vi "DHE_DRV_feedBuffers.vi"(10 "bufsize":u64) -> (0 "error out":errorcluster)   [LabVIEW 2016]
uses:
  c/lib/libarcDHE.so
panel:
  out "error out 2":errorcluster
  in  "stop":bool
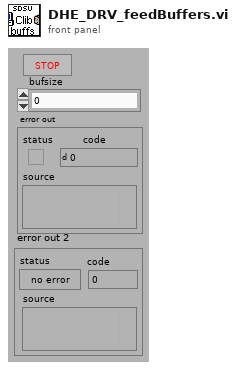
[diagram p1: front panel]
types:
  T1 = cluster{"Name":string, "size (bytes)":u32, "pointer":u32, "Lock":bool}
  T2 = cluster{"Name":string, "size (bytes)":u64, "pointer":u64, "Lock":bool}
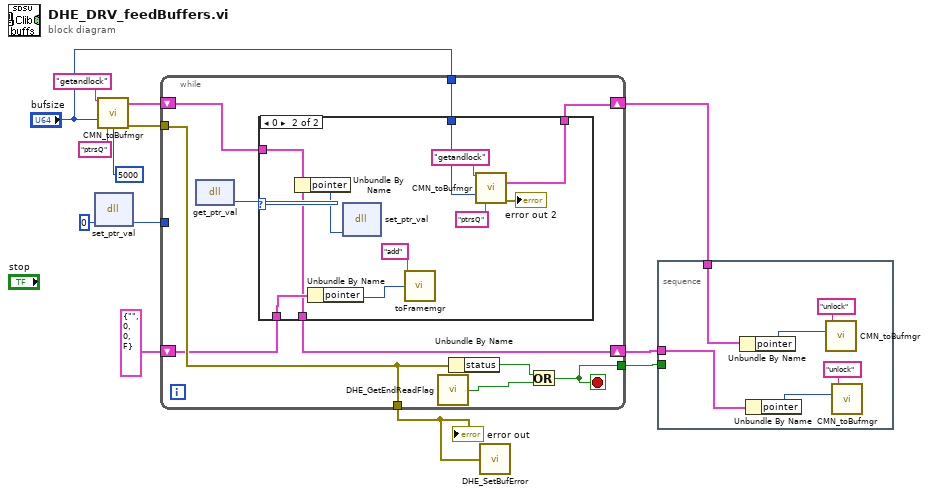
[diagram p0: block diagram]
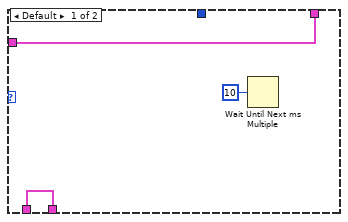
[diagram p2: hidden frame]
diagram:
  n1 = dll-call lib="home/simager/panview/PAN/Modules/SDSU/private/c/lib/libarcDHE.so" fn="set_ptr_val"("ptr"=u64 0) -> ("ptr"=w9:u64)  [unwired: 3 in, 3 out]
  n2 = call "CMN_toBufmgr.vi"("command"="getandlock", "bufsize"="bufsize", "responseQ"="ptrsQ", "ms timeout (-1)"=5000) -> ("buffer"=w11:T2, "error out"=w4:errorcluster)  [unwired: 4 in, 6 out]
  n3 = while {
    tunnel: [w17] -> w1
    tunnel: w4 -> [w17]
    tunnel: [w19] -> w7
    tunnel: "bufsize" -> [w20]
    tunnel: w9 -> [_]
    shift-left: T1 {"Name"="", "size (bytes)"=0, "pointer"=0, "Lock"=FALSE} ("buffer") -> [w16]
    shift-right: [w15] -> w6
    shift-left: w11 -> [w22]
    shift-right: [w21] -> w3
    stop <- w19 stop-if-true
    n4 = dll-call lib="home/simager/panview/PAN/Modules/SDSU/private/c/lib/libarcDHE.so" fn="get_ptr_val"() -> ("return type"=w23:u64)  [unwired: 3 in, 2 out]
    n5 = case shown="0" w23 {
      tunnel: w22 -> [w25 w28]
      tunnel: [w25 w33] -> w21
      tunnel: w20 -> [_ w30]
      tunnel: w16 -> [w24 w29]
      tunnel: [w24 w28] -> w15
      frame Default {
        n6 = Wait Until Next ms Multiple(millisecond multiple=u32 10) -> ()  [unwired: 1 out]
      }
      frame 0 {
        n7 = Unbundle By Name(w28) -> ("pointer"=w36:u64)
        n8 = Unbundle By Name(w29) -> ("pointer"=w31:u64)
        n9 = dll-call lib="home/simager/panview/PAN/Modules/SDSU/private/c/lib/libarcDHE.so" fn="set_ptr_val"("ptr"=w36) -> ()  [unwired: 3 in, 4 out]
        n10 = call "toFramemgr.vi"("command"="add", "bufpointer"=w31) -> ()  [unwired: 7 in, 7 out]
        n11 = call "CMN_toBufmgr.vi"("command"="getandlock", "bufsize"=w30, "responseQ"="ptrsQ") -> ("buffer"=w33:T2, "error out"=→"error out 2":errorcluster)  [unwired: 5 in, 6 out]
      }
    }
    n12 = call "DHE_GetEndReadFlag.vi"() -> ("DHE_read_ended"=w14:bool)  [unwired: 9 out]
    n13 = Unbundle By Name(w17) -> ("status"=w18:bool)
    n14 = Or(x=w18, y=w14) -> (x .or. y?=w19:bool)
  }
  "error out" <- w1
  n15 = call "DHE_SetBufError.vi"("DHE_BufError"=w1) -> ()  [unwired: 9 out]
  n16 = stacked-sequence {
    tunnel: w7 -> [_]
    tunnel: w6 -> [w37]
    tunnel: w3 -> [w42]
    frame #0 {
      n17 = Unbundle By Name(w42) -> ("pointer"=w40:u64)
      n18 = Unbundle By Name(w37) -> ("pointer"=w39:u64)
      n19 = call "CMN_toBufmgr.vi"("command"="unlock", "bufpointer"=w40) -> ()  [unwired: 6 in, 8 out]
      n20 = call "CMN_toBufmgr.vi"("command"="unlock", "bufpointer"=w39) -> ()  [unwired: 6 in, 8 out]
    }
  }
